vi "LTVDiffDriveCtrl_Execute.vi"(5 "LTV_DiffDriveCtrl_Model":T1={"Track Width"=0.2, "Diff_Drive_Linear_System"={"m_A"=[], "m_B"=[], "m_C"=[], "m_D"=[], "States"=0, "Inputs"=0, "Outputs"=0}, "LTV_DiffDriveCtrl_Control"={"Max left vel ctrl effort V"=12.0, "Desired Heading Ctrl Tol Rad"=0.06, "Desired Y Pos Meas Tol M"=0.125, "Desired X Pos Ctrl Tol M"=0.125, "Desired Left Vel Ctrl Tol M/S"=0.1, "Desired Right Vel Ctrl Tol M/S"=0.1, "Max right vel ctrl effort V"=12.0}, "LTV_DiffDriveCtrl_Tolerance"={"Max Heading Tolerance Rad"=0.2, "Max X Tolerance M"=0.0625, "Max Y Tolerance M"=0.125, "Max Left Vel Tol M/S"=0.2, "Max Right Vel Tol M/S"=0.2}, "dT Sec"=0.02} {"LTV_DiffDriveCtrl_Tolerance"."Max Right Vel Tol M/S" format="%#_13g"; "LTV_DiffDriveCtrl_Tolerance"."Max Left Vel Tol M/S" format="%#_13g"; "LTV_DiffDriveCtrl_Tolerance"."Max Y Tolerance M" format="%#_13g"; "LTV_DiffDriveCtrl_Tolerance"."Max X Tolerance M" format="%#_13g"; "LTV_DiffDriveCtrl_Tolerance"."Max Heading Tolerance Rad" format="%#_13g"; "LTV_DiffDriveCtrl_Control"."Max right vel ctrl effort V" format="%#_13g"; "LTV_DiffDriveCtrl_Control"."Desired Right Vel Ctrl Tol M/S" format="%#_13g"; "LTV_DiffDriveCtrl_Control"."Desired Left Vel Ctrl Tol M/S" format="%#_13g"; "LTV_DiffDriveCtrl_Control"."Desired X Pos Ctrl Tol M" format="%#_13g"; "LTV_DiffDriveCtrl_Control"."Desired Y Pos Meas Tol M" format="%#_13g"; "LTV_DiffDriveCtrl_Control"."Desired Heading Ctrl Tol Rad" format="%#_13g"; "LTV_DiffDriveCtrl_Control"."Max left vel ctrl effort V" format="%#_13g"; "Track Width" format="%#_13g"}, 6 "Right Velocity":dbl, 7 "RefPose":T6={"TRANSLATION"={"X"=0.0, "Y"=0.0}, "ROTATION"={"VALUE"=0.0, "COS"=1.0, "SIN"=0.0}} {"ROTATION"."SIN" format="%13.4f"; "ROTATION"."COS" format="%13.4f"; "ROTATION"."VALUE" format="%13.4f"; "TRANSLATION"."Y" format="%14.3f"; "TRANSLATION"."X" format="%14.3f"}, 8 "Left Velocity":dbl, 9 "CurrentPose":T6={"TRANSLATION"={"X"=0.0, "Y"=0.0}, "ROTATION"={"VALUE"=0.0, "COS"=1.0, "SIN"=0.0}} {"ROTATION"."SIN" format="%13.4f"; "ROTATION"."COS" format="%13.4f"; "ROTATION"."VALUE" format="%13.4f"; "TRANSLATION"."Y" format="%14.3f"; "TRANSLATION"."X" format="%14.3f"}, 10 "Ref Right Velocity":dbl, 11 "Ref Left Velocity":dbl) -> (0 "Error":bool, 1 "At Reference":bool, 2 "Right Motor Dmd":dbl, 3 "Left Motor Dmd":dbl, 4 "out LTV_DiffDrive_CONTROLLER":T9)   [LabVIEW 2019, in "Trajectory_Library.lvlib"]
doc: "The linear time-varying (LTV) differential drive controller has a similar form to the LQR, but the model used to compute the controller gain is the nonlinear model linearized around the drivetrain's current state. We precomputed gains for important places in our state-space, then interpolated between them with a look up table (LUT) to save computational resources.Filters the provided voltages to limit a differential drive's linear and angular acceleration.\n\nThis LabVIEW single call function creates and executes the LTV Diff Drive controller. \n\nThe input linear system is defined as:\n - states\n - left velocity (m/s)\n - right velocity (m/s)\n - inputs\n - left voltage (volts)\n - right voltage(volts)\n - outputs\n - left velocity (m/s)\n - right velocity (m/s)\n\n\n\nInputs:\n - LTVDiffDriveCtrl Model -- cluster -- Packed data used to construct the LTV Diff Drive control system.\n - Ref Pose -- Pose2d -- The desired pose setpoint. (Meters, Radians)\n - Ref Left Velocity -- double -- The desired left velocity (Meters/sec)\n - Ref Right Velocity -- double -- The desired right velocity (Meters/sec)\n - Current Pose -- Pose2d -- The current pose. (Meters, Radians)\n - Left Velocity -- double -- The current left velocity (Meters/sec)\n - Right Velocity -- double -- The current right velocity (Meters/sec)\n\nOutputs:\n - Left Motor Dmd -- double -- Left wheel motor demand (+/- 1.0)\n - Right Motor Dmd -- double -- Left wheel motor demand (+/- 1.0)\n - At Reference -- boolean -- If TRUE, the current position is within the tolerance.\n - Error -- boolean -- If TRUE, an error occured.\n - out LTV DiffDriveCtrl -- cluster -- Internal data structure."
uses:
  Trajectory_Library.lvlib
  TypeDef/LTV_DIFF_DRIVE_CTRL.ctl
  TypeDef/FUNCTION_GENERATOR_MATRIX.ctl
  <vilib>/Analysis/Matrix/Datatypes/RealMatrix.ctl
  TypeDef/POSE2D.ctl
  TypeDef/TRANSLATION2D.ctl
  TypeDef/ROTATION2D.ctl
  TypeDef/LTV_DIFF_DRIVE_CTRL_MODEL_PARAMS.CTL
  TypeDef/LINEAR_SYSTEM.ctl
  TypeDef/LTV_DIFF_DRIVE_CTRL_CONTROL_PARAMS.CTL
  TypeDef/LTV_DIFF_DRIVE_CTRL_TOLERANCE.CTL
  Rotation2d_CreateAngle.vi
  Translation2d_Create.vi
  MatBuilder_Create.vi
  Pose2d_getXYAngle.vi
  <vilib>/Analysis/Matrix/NI_Matrix.lvlib
panel:
  # "<States,States>"
  # "<States,Inputs>"
  # "<Outputs,States>"
  # "<Outputs,Inputs>"
  # "< 5, 1 >"
  # "< 2, 1 >"
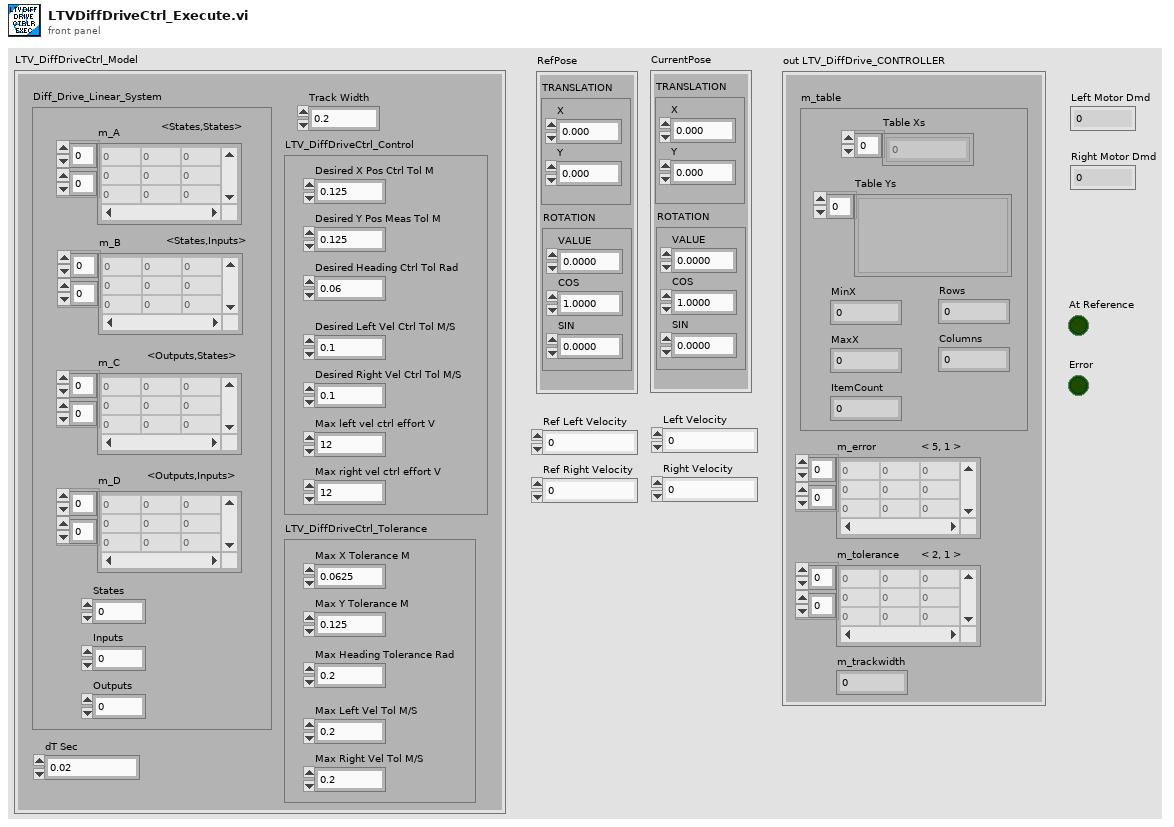
[diagram p1: front panel]
types:
  T1 = typedef "Trajectory_Library.lvlib/LTV_DIFF_DRIVE_CTRL_MODEL_PARAMS.CTL" = cluster{"Track Width":dbl, "Diff_Drive_Linear_System":T2, "LTV_DiffDriveCtrl_Control":T4, "LTV_DiffDriveCtrl_Tolerance":T5, "dT Sec":dbl}
  T2 = typedef "Trajectory_Library.lvlib/LINEAR_SYSTEM.ctl" = cluster{"m_A":T3, "m_B":T3, "m_C":T3, "m_D":T3, "States":i32, "Inputs":i32, "Outputs":i32}
  T3 = typedef "NI_Matrix.lvlib/RealMatrix.ctl" = dbl[][]
  T4 = typedef "Trajectory_Library.lvlib/LTV_DIFF_DRIVE_CTRL_CONTROL_PARAMS.CTL" = cluster{"Max left vel ctrl effort V":dbl, "Desired Heading Ctrl Tol Rad":dbl, "Desired Y Pos Meas Tol M":dbl, "Desired X Pos Ctrl Tol M":dbl, "Desired Left Vel Ctrl Tol M/S":dbl, "Desired Right Vel Ctrl Tol M/S":dbl, "Max right vel ctrl effort V":dbl}
  T5 = typedef "Trajectory_Library.lvlib/LTV_DIFF_DRIVE_CTRL_TOLERANCE.CTL" = cluster{"Max Heading Tolerance Rad":dbl, "Max X Tolerance M":dbl, "Max Y Tolerance M":dbl, "Max Left Vel Tol M/S":dbl, "Max Right Vel Tol M/S":dbl}
  T6 = typedef "Trajectory_Library.lvlib/POSE2D.ctl" = cluster{"TRANSLATION":T7, "ROTATION":T8}
  T7 = typedef "Trajectory_Library.lvlib/TRANSLATION2D.ctl" = cluster{"X":dbl, "Y":dbl}
  T8 = typedef "Trajectory_Library.lvlib/ROTATION2D.ctl" = cluster{"VALUE":dbl, "COS":dbl, "SIN":dbl}
  T9 = typedef "Trajectory_Library.lvlib/LTV_DIFF_DRIVE_CTRL.ctl" = cluster{"m_table":T10, "m_error":T3, "m_tolerance":T3, "m_trackwidth":dbl}
  T10 = typedef "Trajectory_Library.lvlib/FUNCTION_GENERATOR_MATRIX.ctl" = cluster{"Table Xs":dbl[], "Table Ys":variant[], "MinX":dbl, "MaxX":dbl, "ItemCount":i32, "Rows":i32, "Columns":i32}
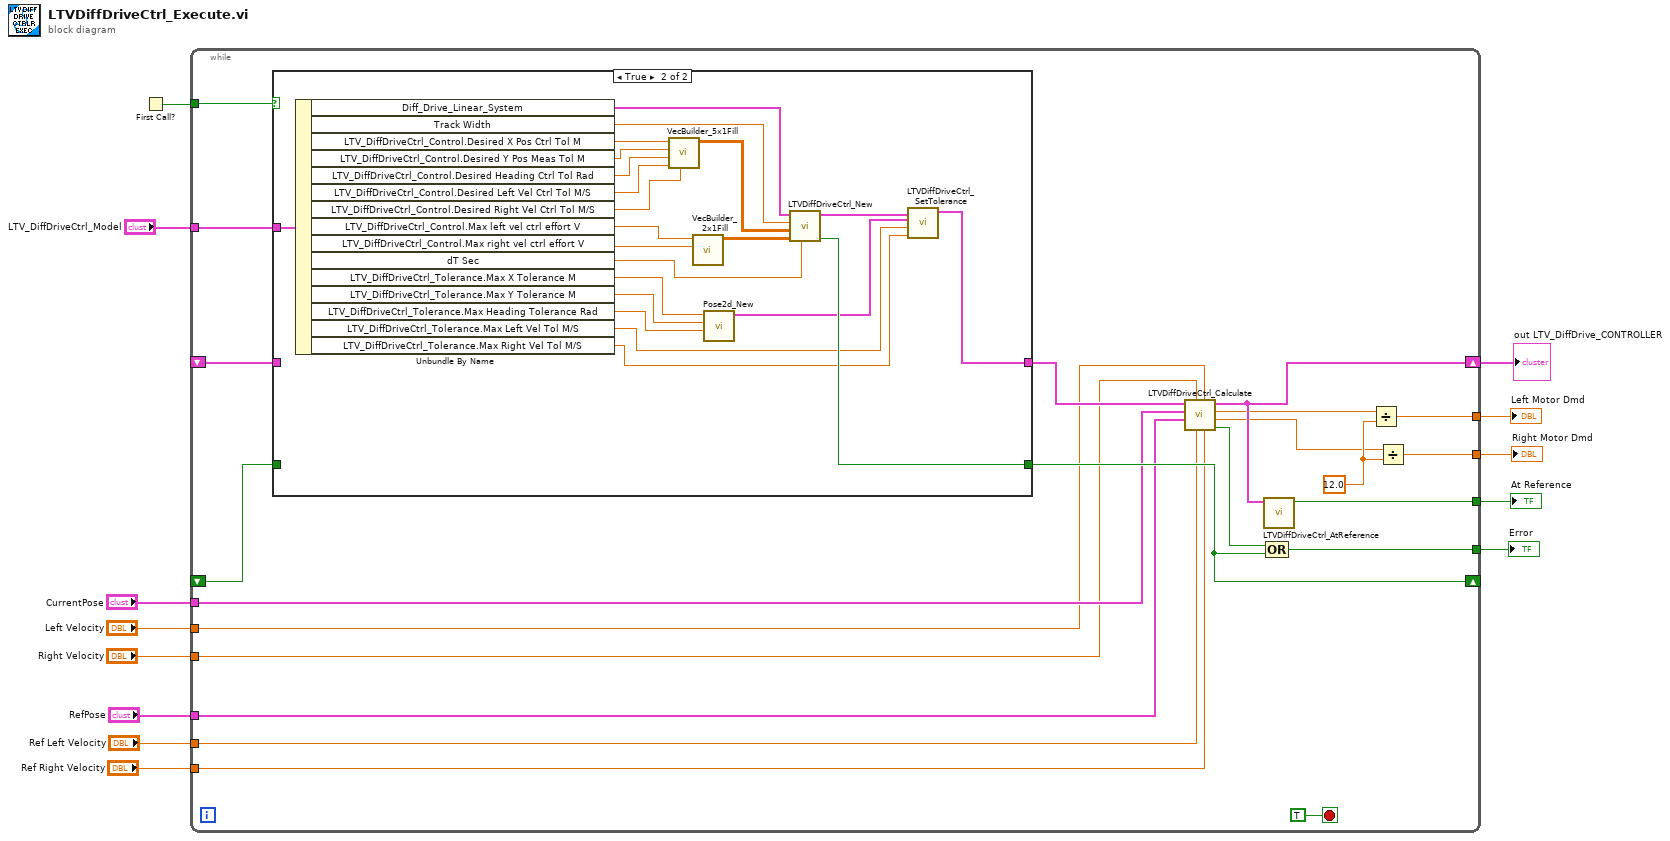
[diagram p0: block diagram]
diagram:
  n1 = First Call?() -> (First Call?: T/F=w11:bool)
  n2 = while {
    shift-right: [w35] -> w7
    shift-left: _ -> [w31]
    tunnel: [w34] -> w13
    tunnel: [w32] -> w12
    tunnel: w11 -> [w30]
    shift-right: [w29] -> _
    shift-left: _ -> [w28]
    tunnel: "CurrentPose" -> [w27]
    tunnel: "RefPose" -> [w26]
    tunnel: "LTV_DiffDriveCtrl_Model" -> [w24]
    tunnel: [w16] -> w6
    tunnel: [w14] -> w5
    tunnel: "Ref Left Velocity" -> [w22]
    tunnel: "Ref Right Velocity" -> [w21]
    tunnel: "Right Velocity" -> [w20]
    tunnel: "Left Velocity" -> [w19]
    stop <- TRUE stop-if-true
    w18 = 12.0 ("y")
    n3 = case shown="True" w30 {
      tunnel: [w37 w59] -> w23
      tunnel: w31 -> [w37 _]
      tunnel: [w36 w57] -> w29
      tunnel: w28 -> [w36 _]
      tunnel: w24 -> [_ w56]
      frame False {
      }
      frame True {
        n4 = Unbundle By Name(w56) -> ("Diff_Drive_Linear_System"=w54:T2, "Track Width"=w53:dbl, "LTV_DiffDriveCtrl_Control.Desired X Pos Ctrl Tol M"=w50:dbl, "LTV_DiffDriveCtrl_Control.Desired Y Pos Meas Tol M"=w49:dbl, "LTV_DiffDriveCtrl_Control.Desired Heading Ctrl Tol Rad"=w48:dbl, "LTV_DiffDriveCtrl_Control.Desired Left Vel Ctrl Tol M/S"=w47:dbl, "LTV_DiffDriveCtrl_Control.Desired Right Vel Ctrl Tol M/S"=w46:dbl, "LTV_DiffDriveCtrl_Control.Max left vel ctrl effort V"=w44:dbl, "LTV_DiffDriveCtrl_Control.Max right vel ctrl effort V"=w43:dbl, "dT Sec"=w45:dbl, "LTV_DiffDriveCtrl_Tolerance.Max X Tolerance M"=w42:dbl, "LTV_DiffDriveCtrl_Tolerance.Max Y Tolerance M"=w41:dbl, "LTV_DiffDriveCtrl_Tolerance.Max Heading Tolerance Rad"=w40:dbl, "LTV_DiffDriveCtrl_Tolerance.Max Left Vel Tol M/S"=w39:dbl, "LTV_DiffDriveCtrl_Tolerance.Max Right Vel Tol M/S"=w38:dbl)
        n5 = call "VecBuilder_5x1Fill.vi"("R4"=w46, "R3"=w47, "R2"=w48, "R1"=w49, "R0"=w50) -> ("output matrix"=w51:T3)  [unwired: 6 in]
        n6 = call "VecBuilder_2x1Fill.vi"("R1"=w43, "R0"=w44) -> ("output matrix"=w52:T3)  [unwired: 9 in]
        n7 = call "Pose2d_New.vi"("Heading"=w40, "Y"=w41, "X"=w42) -> ("out POSe"=w55:T6)  [unwired: 8 in]
        n8 = call "LTVDiffDriveCtrl_New.vi"("dT"=w45, "Relms"=w52, "Qelms"=w51, "TrackWidth"=w53, "Plant"=w54) -> ("Error"=w57:bool, "DiffDriveCtrl"=w58:T9)  [unwired: 5 in]
        n9 = call "LTVDiffDriveCtrl_SetTolerance.vi"("RightVelTolerance"=w38, "LeftVelTolerance"=w39, "PoseTolerance"=w55, "in LTV_DIFF_DRIVE_CONTROLLER"=w58) -> ("out LTV_DIFF_DRIVE_CONTROLLER"=w59:T9)  [unwired: 7 in]
      }
    }
    n10 = call "LTVDiffDriveCtrl_Calculate.vi"("Ref Right Velocity"=w21, "Left Velocity"=w19, "Ref Left Velocity"=w22, "Right Velocity"=w20, "RefPose"=w26, "CurrentPose"=w27, "in LTVDiffDriveCtrl"=w23) -> ("Error"=w33:bool, "Right Voltage"=w15:dbl, "Left Voltage"=w17:dbl, "out LTVDiffDriveCtrl"=w35:T9)  [unwired: 1 in]
    n11 = call "LTVDiffDriveCtrl_AtReference.vi"("LTV_DIFF_DRIVE_CTRL"=w35) -> ("At Reference"=w34:bool)  [unwired: 10 in]
    n12 = Compound Arithmetic op=OR(w33, w29) -> (w32:bool)
    n13 = Divide(x=w17, y=w18) -> (x/y=w16:dbl)
    n14 = Divide(x=w15, y=w18) -> (x/y=w14:dbl)
  }
  "out LTV_DiffDrive_CONTROLLER" <- w7
  "Error" <- w12
  "At Reference" <- w13
  "Left Motor Dmd" <- w6
  "Right Motor Dmd" <- w5
